vi "VG_OP400.vi"() -> ()   [LabVIEW 2020]
panel:
  out "Sealing max":dbl
  out "Sealing min":dbl
  out "Humidity max":dbl
  out "Humiditymin":dbl
  out "Temp max":dbl
  out "Temp min":dbl
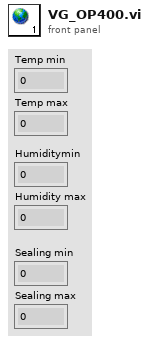
[diagram p1: front panel]
diagram:
